vi "Main2.vi"() -> ()   [LabVIEW 2019]
panel:
  in  "Tab Control":enum32{"Page 1", "Page 2"}(tab)
  out "Waveform Chart 2":cluster{dbl, dbl, dbl}(graph)
  in  "VISA resource name":refnum<visa-resource-name>="COM3"
  in  "termination char\n(0xA = '\\n' = LF)":u8=13 format="%.0x"
  in  "Recieve Data":bool
  out "Waveform Chart 3":dynamicdata(graph)
  in  "device name":tag="PXI1Slot2"
  in  "timeout (s)":dbl=10.0 format="%0.2f"
  in  "stop":bool
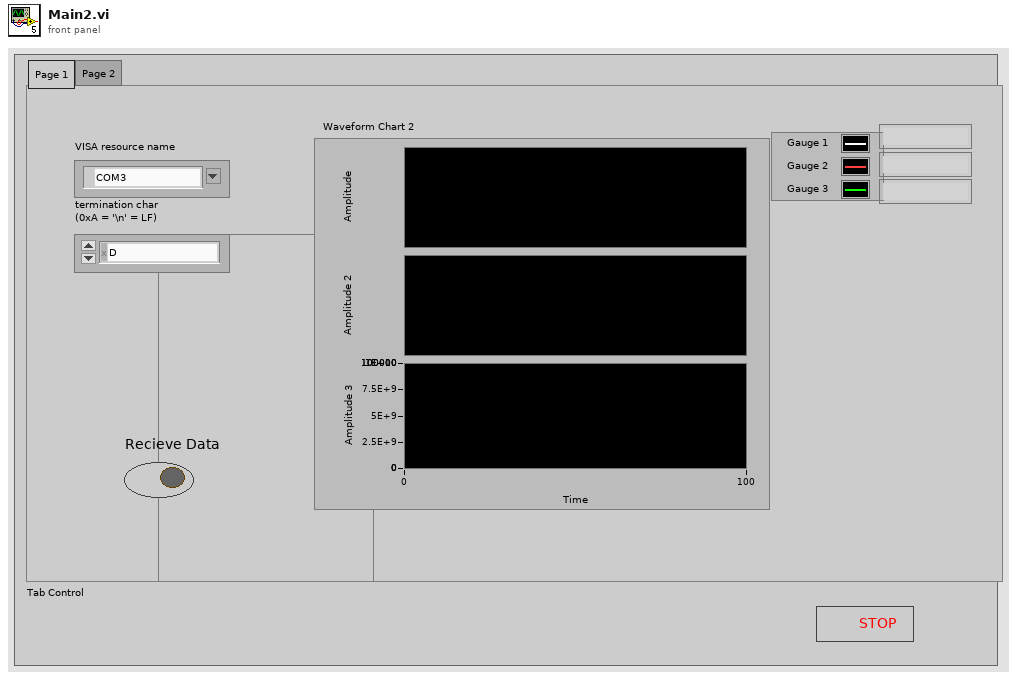
[diagram p1: front panel]
types:
  T1 = enum16{"open", "replace", "create", "open or create", "replace or create", "replace or create with confirmation"}
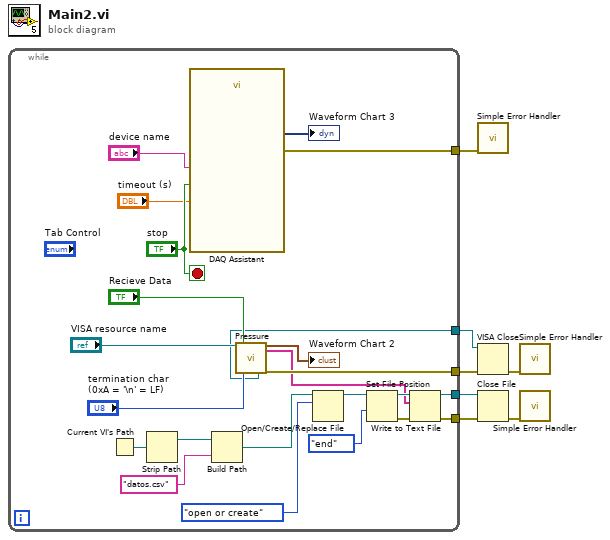
[diagram p0: block diagram]
diagram:
  n1 = while {
    tunnel: [w26] -> w7
    tunnel: [w25] -> w6
    tunnel: [w14] -> w3
    tunnel: [w13] -> w2
    tunnel: [w11] -> w1
    stop <- "stop" stop-if-true
    n2 = Current VI's Path() -> (path=w21:path)
    n3 = Strip Path(path=w21) -> (stripped path=w22:path)  [unwired: 1 out]
    n4 = call "DAQ Assistant"("timeout (s)"="timeout (s)", "stop (T)"="stop", "device name"="device name") -> ("data"=→"Waveform Chart 3":dynamicdata, "error out"=w11:errorcluster)  [unwired: 14 in, 1 out]
    n5 = Build Path(base path=w22, name or relative path="datos.csv") -> (appended path=w23:path)
    n6 = call "Pressure.vi"("VISA resource name"="VISA resource name", "Recieve Data"="Recieve Data", "termination char\n(0xA = '\\n' = LF)"="termination char\n(0xA = '\\n' = LF)") -> ("VISA resource name out"=w25:refnum<visa-resource-name>, "output cluster"=→"Waveform Chart 2":cluster{dbl, dbl, dbl}, "output array"=w15:string[], "error out"=w26:errorcluster)  [unwired: 10 in, 3 out]
    n7 = Open/Create/Replace File(file path (use dialog)=w23, operation (0:open)=T1."open or create") -> (refnum out=w24:refnum<file>)  [unwired: 4 in, 2 out]
    n8 = Set File Position(refnum=w24, from (0:start)=enum16{"start", "end", "current"}."end") -> (refnum out=w17:refnum<file>, error out=w16:errorcluster)  [unwired: 2 in]
    n9 = Write to Text File(file (use dialog)=w17, text=w15, error in=w16) -> (refnum out=w14:refnum<file>, error out=w13:errorcluster)  [unwired: 1 in, 1 out]
  }
  n10 = call <vilib>:"Simple Error Handler.vi"("error in (no error)"=w1) -> ()  [unwired: 4 in, 5 out]
  n11 = VISA Close(VISA resource name=w6, error in (no error)=w7) -> (error out=w5:errorcluster)
  n12 = Close File(refnum=w3, error in=w2) -> (error out=w4:errorcluster)  [unwired: 1 out]
  n13 = call <vilib>:"Simple Error Handler.vi"("error in (no error)"=w5) -> ()  [unwired: 4 in, 5 out]
  n14 = call <vilib>:"Simple Error Handler.vi"("error in (no error)"=w4) -> ()  [unwired: 1 in, 8 out]
